vi "Close Hardware Session.vi"(8 "error in":errorcluster, 11 "hardware handles":T1) -> (0 "error out":errorcluster)   [LabVIEW 2020, in "Ballard MIL-STD-1553 Engine.lvlib" / "Custom Device.lvlib"]
uses:
  Custom Device.lvlib
  Hardware Handles.ctl
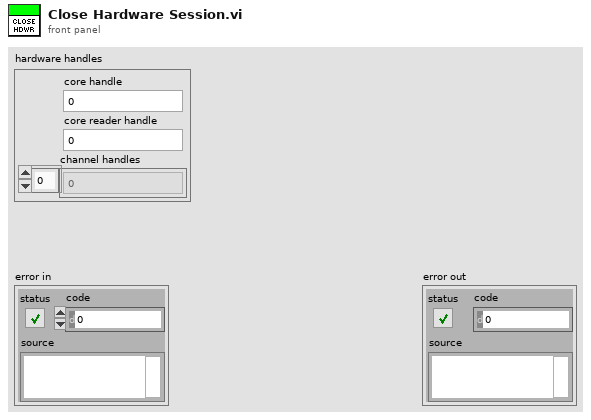
[diagram p1: front panel]
types:
  T1 = typedef "Ballard MIL-STD-1553 Engine.lvlib/Custom Device.lvlib/Hardware Handles.ctl" = cluster{"core handle":u64, "core reader handle":u64, "channel handles":u64[]}
  T2 = cluster{"core handle":u64, "core reader handle":u64}
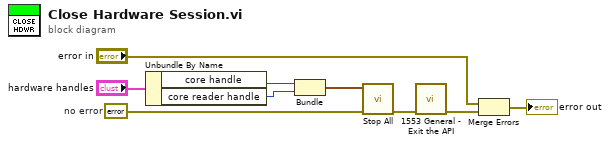
[diagram p0: block diagram]
diagram:
  w6 = errorcluster {"status"=FALSE, "code"=0, "source"=""}  # no error
  n1 = Unbundle By Name("hardware handles") -> ("core handle"=w3:u64, "core reader handle"=w2:u64)
  n2 = Bundle("core handle"=w3, "core reader handle"=w2) -> (w1:T2)  [unwired: 1 in]
  n3 = call "Stop All.vi"("Error In"=w6, "Module Reference"=w1) -> ("Error Out"=w7:errorcluster)  [unwired: 8 in, 1 out]
  n4 = call <instrlib>:"1553 General - Exit the API.vi"("Error In (none)"=w7) -> ("Error Out"=w5:errorcluster)  [unwired: 10 in]
  n5 = Merge Errors("error in", w5) -> (→"error out":errorcluster)
